vi "DAQmx Create Channel (AI-Sound Pressure-Microphone).vi"(0 "task in":refnum<k21>, 1 "maximum sound pressure level":dbl=100.0 format="%0.2f", 3 "input terminal configuration":i32(ring)=-1 items=["default"=-1, "RSE"=10083, "NRSE"=10078, "Differential"=10106, "Pseudodifferential"=12529], 5 "physical channels":tag, 6 "current excitation source":i32(ring)=10200 items=["Internal"=10200, "External"=10167, "None"=10230], 7 "name to assign":string, 8 "current excitation value":dbl=0.004, 9 "units":i32(ring)=10081 items=["Pascals"=10081, "From Custom Scale"=10065], 11 "error in":errorcluster, 12 "custom scale name":tag, 13 "microphone sensitivity":dbl=10.0) -> (4 "task out":refnum<k21>, 15 "error out":errorcluster)   [LabVIEW 2020]
doc: "Creates channel(s) that use a microphone to measure sound pressure."
uses:
  nilvaiu.dll
panel:
  # "input limits"
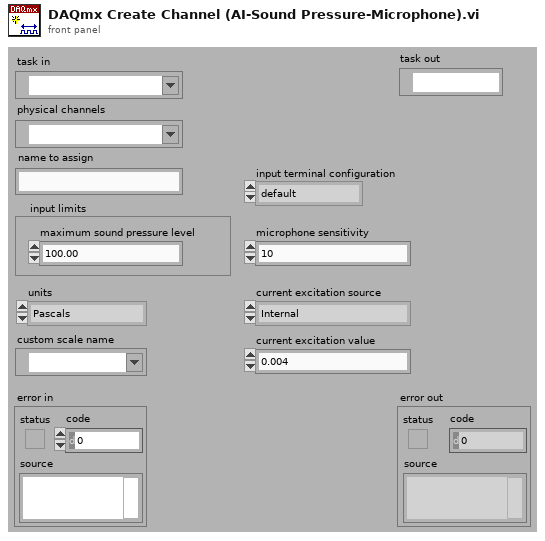
[diagram p1: front panel]
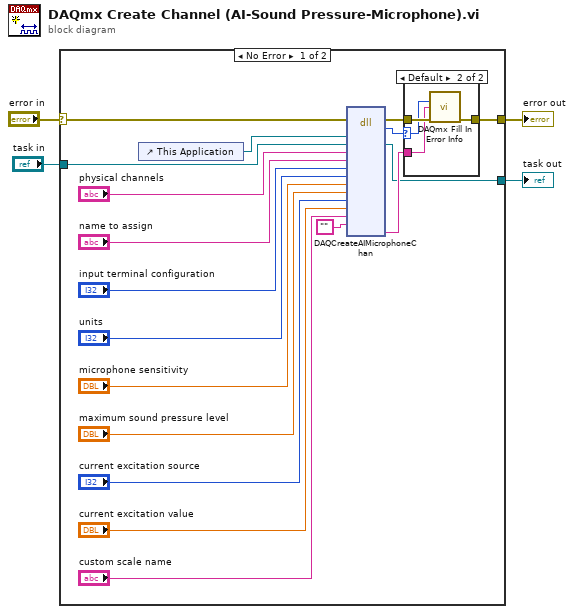
[diagram p0: block diagram]
diagram:
  n1 = case shown="No Error" "error in" {
    selector: "error in" -> [w16 w29]
    tunnel: [w17 w29] -> w2
    tunnel: "task in" -> [w15 w28]
    tunnel: [w14 w28] -> w1
    frame No Error {
      n2 = control-ref of="This Application"() -> (w19:refnum<vi>)
      n3 = dll-call lib="nilvaiu.*" fn="DAQCreateAIMicrophoneChan"(error in=w16, "lvAppRef"=w19, "refObjPtr"=w15, "physicalChannelName"="physical channels", "channelNameIn"="name to assign", "terminalConfig"="input terminal configuration", "units"="units", "micSensitivity"="microphone sensitivity", "maxSndPressLevel"="maximum sound pressure level", "currExcSrc"="current excitation source", "currExcVal"="current excitation value", "customScaleName"="custom scale name", "channelNamesOut"="") -> (error out=w22:errorcluster, "return type"=w21:i32, "refObjPtr"=w14:refnum<k21>, "extendedErrorInfo"=w20:string)  [unwired: 14 in, 1 out]
      n4 = case shown="Default" w21 {
        selector: w21 -> [_ w25]
        tunnel: w22 -> [w23 w27]
        tunnel: [w23 w26] -> w17
        tunnel: w20 -> [_ w24]
        frame 0 {
        }
        frame Default {
          n5 = call "DAQmx Fill In Error Info.vi"("status code"=w25, "extended error info"=w24, "error in"=w27) -> ("error out"=w26:errorcluster)  [unwired: 1 in, 11 out]
        }
      }
    }
    frame Error {
    }
  }
  "error out" <- w2
  "task out" <- w1
